vi "Test Write (String).vi"() -> ()   [LabVIEW 2020, in "sqlite3.lvlib"]
uses:
  sqlite3.lvlib
  sqlite/VIs/open v2.vi
  sqlite/VIs/prepare v2.vi
  sqlite/VIs/step.vi
  sqlite/VIs/column count.vi
  compound/Column.vi
  compound/Resolve Result Type.vi
  sqlite/VIs/finalize.vi
  sqlite/VIs/close v2.vi
  sqlite/subvi/Error Converter (ErrCode or Status).vi
  sqlite/VIs/column text.vi
  sqlite/VIs/column bytes.vi
  sqlite/VIs/column blob.vi
  utilities/MoveBlock.vi
  sqlite/VIs/column type.vi
  sqlite/VIs/errstr.vi
panel:
  out "Query Result 2":string[][](array[string])
  out "Query Result":string[][](array[string])
  out "error out":errorcluster
  in  "database in":path=path "C:/labview/sqlite_dbManager/test database/newtest.db"
  in  "error in (no error)":errorcluster
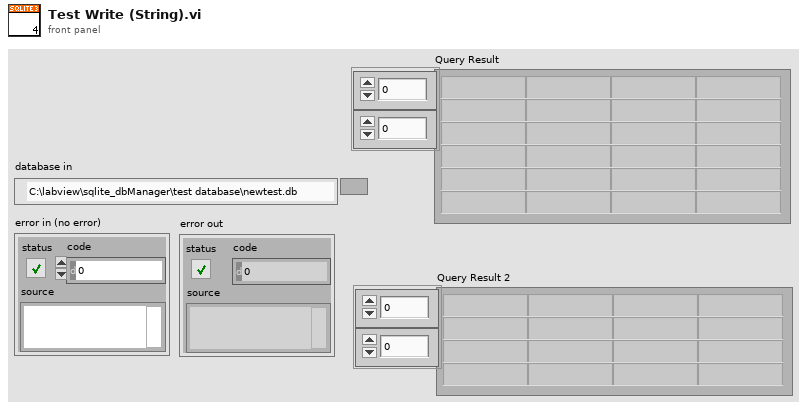
[diagram p1: front panel]
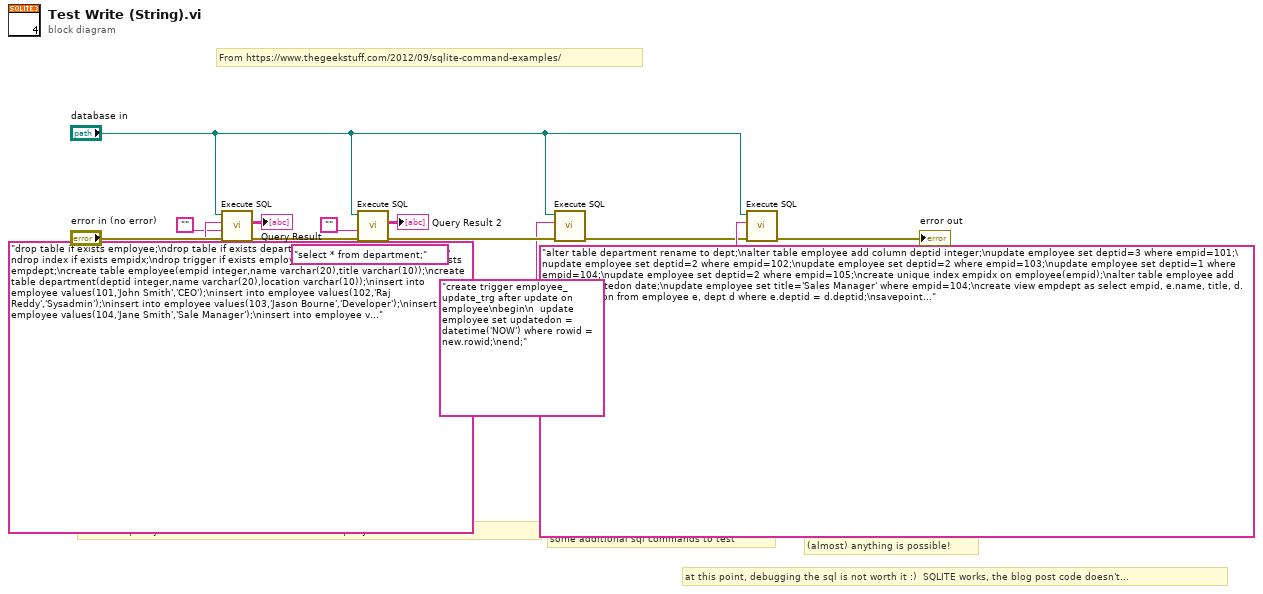
[diagram p0: block diagram]
diagram:
  # "at this point, debugging the sql is not worth it :)  SQLITE works, the blog post code doesn't..."
  # "(almost) anything is possible!"
  # "some additional sql commands to test"
  # "From https://www.thegeekstuff.com/2012/09/sqlite-command-examples/"
  # "execute sql only returns last statement in a list.  new query for new return value"
  # "create test table"
  n1 = call "Execute SQL.vi"("error in (no error)"="error in (no error)", "[disabled] return type (string)"="", "sql (string)"="drop table if exists employee;\ndrop table if exists department;\ndrop table if exists dept;\ndrop index if exists empidx;\ndrop trigger if exists employee_update_trg;\ndrop view if exists empdept;\ncreate table employee(empid integer,name varchar(20),title varchar(10));\ncreate table department(deptid integer,name varchar(20),location varchar(10));\ninsert into employee values(101,'John Smith','CEO');\ninsert into employee values(102,'Raj Reddy','Sysadmin');\ninsert into employee values(103,'Jason Bourne','Developer');\ninsert into employee values(104,'Jane Smith','Sale Manager');\ninsert into employee values(105,'Rita Patel','DBA');\ninsert into department values(1,'Sales','Los Angeles');\ninsert into department values(2,'Technology','San Jose');\ninsert into department values(3,'Marketing','Los Angeles');\nselect * from employee;", "database in"="database in") -> ("error out"=w13:errorcluster, "Query Result"=→"Query Result":string[][])  [unwired: 6 in]
  n2 = call "Execute SQL.vi"("error in (no error)"=w13, "[disabled] return type (string)"="", "sql (string)"="select * from department;", "database in"="database in") -> ("error out"=w3:errorcluster, "Query Result"=→"Query Result 2":string[][])  [unwired: 6 in]
  n3 = call "Execute SQL.vi"("error in (no error)"=w3, "sql (string)"="create trigger employee_update_trg after update on employee\nbegin\n  update employee set updatedon = datetime('NOW') where rowid = new.rowid;\nend;", "database in"="database in") -> ("error out"=w2:errorcluster)  [unwired: 7 in, 1 out]
  n4 = call "Execute SQL.vi"("error in (no error)"=w2, "sql (string)"="alter table department rename to dept;\nalter table employee add column deptid integer;\nupdate employee set deptid=3 where empid=101;\nupdate employee set deptid=2 where empid=102;\nupdate employee set deptid=2 where empid=103;\nupdate employee set deptid=1 where empid=104;\nupdate employee set deptid=2 where empid=105;\ncreate unique index empidx on employee(empid);\nalter table employee add column updatedon date;\nupdate employee set title='Sales Manager' where empid=104;\ncreate view empdept as select empid, e.name, title, d.name, location from employee e, dept d where e.deptid = d.deptid;\nsavepoint major;\ninsert into dept values(4,'HR','Los Angeles');\ninsert into dept values(5,'Finance','San Jose');\ndelete from dept where deptid=1;\nrollback to savepoint major;\nrelease savepoint major;", "database in"="database in") -> ("error out"=→"error out":errorcluster)  [unwired: 7 in, 1 out]
